vi "Thermo Gas Conc Read Single Instr. (SubVI).vi"(7 "remote port":u16=502, 8 "Error In":errorcluster, 9 "MBAP Header":cluster{"Transaction ID":u16, "Unit ID":u8}={"Transaction ID"=0, "Unit ID"=42}, 10 "Quantity NOx":u16=6, 11 "IP Address":string="192.168.1.201") -> (0 "error out":errorcluster, 3 "Data Out":T1(array[cluster]))   [LabVIEW 2011]
uses:
  <vilib>/Utility/error.llb/DialogType.ctl
  <vilib>/NI Modbus.llb/MB Ethernet Master Query Read Holding Registers (poly).vi
panel:
  in  "Starting Address":u16
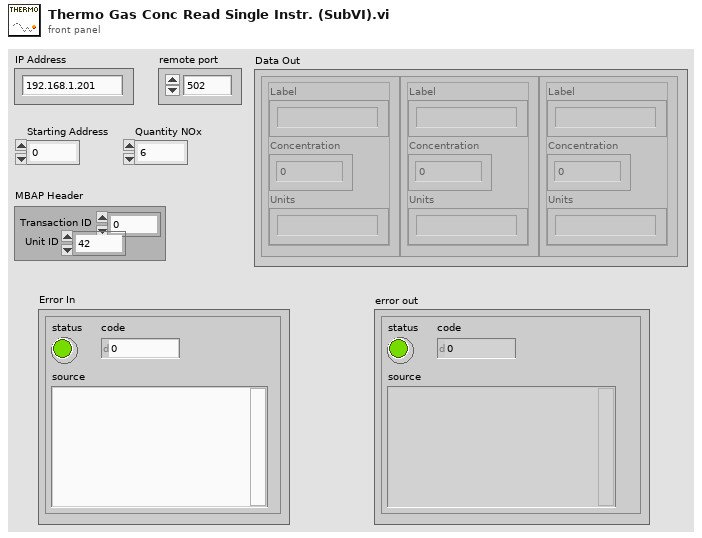
[diagram p1: front panel]
types:
  T1 = cluster{"Label":string, "Concentration":sgl, "Units":string}[]
  T2 = typedef "DialogType.ctl" = u16
  T3 = cluster{"Label":string, "Concentration":sgl, "Units":string}
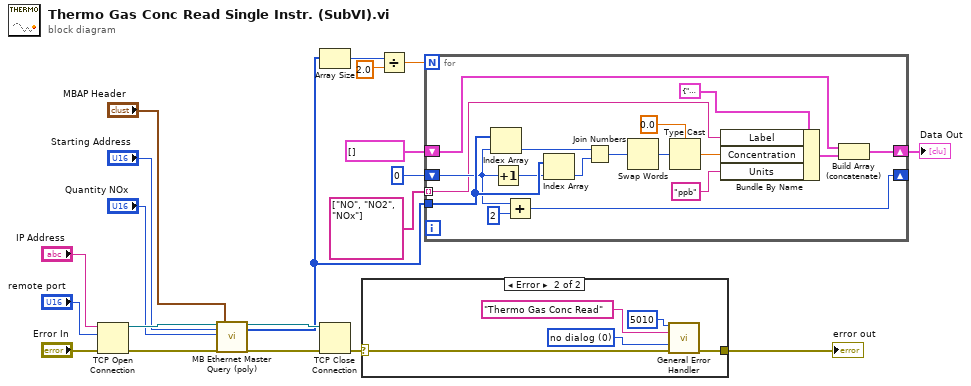
[diagram p0: block diagram]
diagram:
  n1 = TCP Open Connection(address="IP Address", remote port or service name="remote port", error in (no error)="Error In") -> (connection ID=w18:refnum<k5>, error out=w17:errorcluster)  [unwired: 2 in]
  n2 = call-poly <vilib>:"MB Ethernet Master Query (poly).vi"("TCP Connection Refnum in"=w18, "Starting Address"="Starting Address", "Quantity"="Quantity NOx", "error in"=w17, "MBAP Header"="MBAP Header") -> ("TCP Connection Refnum (dup)"=w20:refnum<k5>, "Holding Registers"=w8:u16[], "error out"=w19:errorcluster)  [unwired: 11 in, 1 out]
  n3 = Array Size(array=w8) -> (size(s)=w13:i32)
  n4 = TCP Close Connection(connection ID=w20, error in (no error)=w19) -> (error out=w2:errorcluster)  [unwired: 1 in, 1 out]
  n5 = case shown="Error" w2 {
    selector: w2 -> [w21 w23]
    tunnel: [w21 w22] -> w1
    frame No Error {
    }
    frame Error {
      w24 = T2 0 items=["no dialog", "OK message", "continue or stop message", "OK message + warnings", "continue/stop + warnings"] ("type of dialog (OK msg:1)")
      n6 = call <vilib>:"General Error Handler.vi"("[error code] (0)"=5010, "[error source] (\" \")"="Thermo Gas Conc Read" ("[error source] (\" \")"), "type of dialog (OK msg:1)"=w24, "error in (no error)"=w23) -> ("error out"=w22:errorcluster)  [unwired: 7 in, 4 out]
    }
  }
  "error out" <- w1
  n7 = Divide(x=w13, y=2.0) -> (x/y=w12:dbl)
  n8 = for {
    N: w12 -> [_]
    tunnel: w8 -> [w43]
    shift-right: [w29] -> w9
    shift-left: T1 [] -> [w28]
    shift-right: [w35] -> _
    shift-left: 0 -> [w33]
    tunnel: string[] ["NO", "NO2", "NOx"] -> [w27] mode=indexing
    n9 = Index Array(array=w43, index=w33) -> (element=w40:u16)
    n10 = Increment(x=w33) -> (x+1=w32:i32)
    n11 = Add(x=w33, y=2) -> (x+y=w35:i32)
    n12 = Index Array(array=w43, index=w32) -> (element=w39:u16)
    n13 = Join Numbers(hi=w40, lo=w39) -> ((hi.lo)=w41:u32)
    n14 = Swap Words(1:w41) -> (0:w38:u32)
    n15 = Type Cast(type=sgl 0.0, x=w38) -> (*(type *) &x=w37:sgl)
    n16 = Bundle By Name(cluster=T3 {"Label"="", "Concentration"=0.0, "Units"=""}, "Label"=w27, "Concentration"=w37, "Units"="ppb") -> (w31:T3)
    n17 = Build Array (concatenate)(w28, w31) -> (w29:T1)
  }
  "Data Out" <- w9
